vi "Startup.vi"(6 "LabVIEW Web Service":refnum<class "Web Service.lvclass">) -> ()   [LabVIEW 2014]
uses:
  <vilib>/wsapi/Web Service.lvclass
  Controller/Messages/Log Message MSG/Send Log Message MSG.lvclass
  Controller/Controller.lvclass
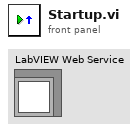
[diagram p1: front panel]
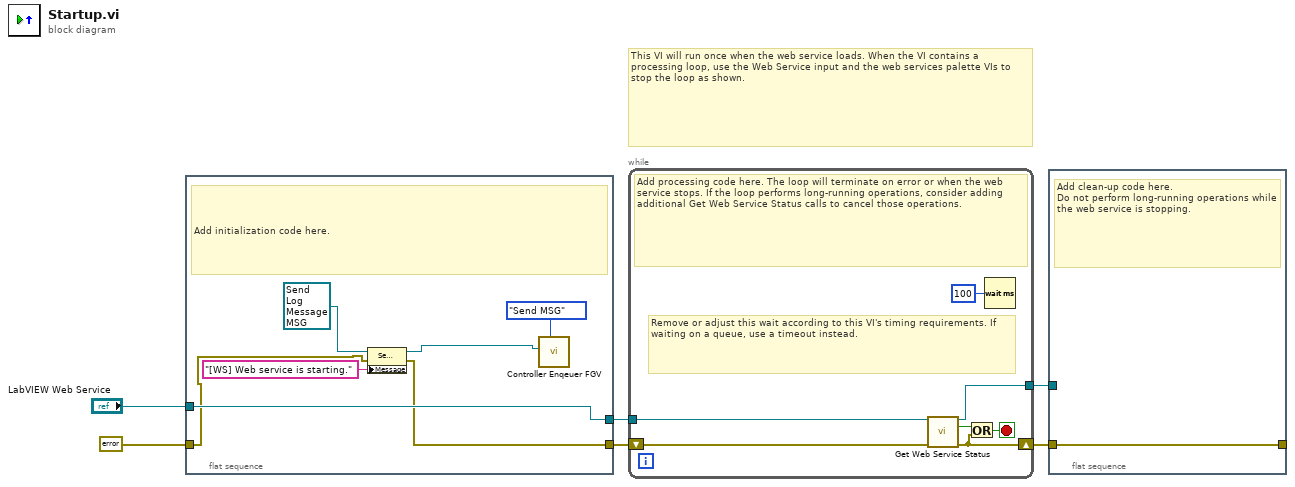
[diagram p0: block diagram]
diagram:
  # "This VI will run once when the web service loads. When the VI contains a processing loop, use the Web Service input and the web services palette VIs to stop the loop as shown."
  n1 = flat-sequence {
    tunnel: "LabVIEW Web Service" -> [w13]
    tunnel: [w13] -> w5
    tunnel: [w7] -> w4
    tunnel: errorcluster {"status"=FALSE, "code"=0, "source"=""} ("error constant") -> [w8]
    frame #0 {
      # "Add initialization code here."
      n2 = property class="Send Log Message MSG.lvclass"(reference=refnum<class "Send Log Message MSG.lvclass"> refnum ("Controller:Send Log Message MSG.lvclass"), error in=w8, "Message"="[WS] Web service is starting.") -> (reference out=w9:refnum<class "Send Log Message MSG.lvclass">, error out=w7:errorcluster)
      n3 = call "Controller Enqeuer FGV.vi"("State"=enum16{"Store", "Send MSG"}."Send MSG", "MSG"=w9) -> ()  [unwired: 9 in, 1 out]
    }
  }
  n4 = while {
    tunnel: w5 -> [w14]
    shift-right: [w17] -> w2
    shift-left: w4 -> [w18]
    tunnel: [w15] -> w1
    stop <- w19 stop-if-true
    # "Remove or adjust this wait according to this VI's timing requirements. If waiting on a queue, use a timeout instead."
    # "Add processing code here. The loop will terminate on error or when the web service stops. If the loop performs long-running operations, consider adding additional Get Web Service Status calls to cancel those operations."
    n5 = call <vilib>:"Get Web Service Status.vi"("LabVIEW Web Service"=w14, "error in (no error)"=w18) -> ("LabVIEW Web Service out"=w15:refnum<class "Web Service.lvclass">, "service stopping?"=w20:bool, "error out"=w17:errorcluster)  [unwired: 11 in]
    n6 = Or(x=w20, y=w17) -> (x .or. y?=w19:bool)
    n7 = Wait (ms)(milliseconds to wait=u32 100) -> ()  [unwired: 1 out]
  }
  n8 = flat-sequence {
    tunnel: [w21] -> _
    tunnel: w2 -> [w21]
    tunnel: w1 -> [_]
    frame #0 {
      # "Add clean-up code here.\nDo not perform long-running operations while the web service is stopping."
    }
  }
